vi "Intensity.vi"(1 "PSD[0]":dbl[](array[numeric])) -> (0 "Intensity":T1)   [LabVIEW 2013]
uses:
  <vilib>/Analysis/5stat.llb/RMS (DBL).vi
  <vilib>/Analysis/NI_AALPro.lvlib
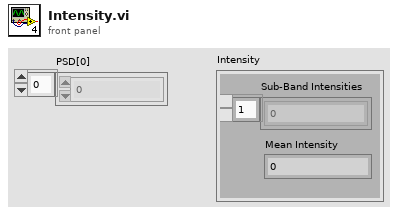
[diagram p1: front panel]
types:
  T1 = cluster{"Sub-Band Intensities":dbl[], "Mean Intensity":dbl}
  T2 = cluster{"1":dbl[], "2":dbl[], "3":dbl[], "4":dbl[], "5":dbl[], "6":dbl[], "7":dbl[]}
  T3 = cluster{"rms value":dbl, "rms value":dbl, "rms value":dbl, "rms value":dbl, "rms value":dbl, "rms value":dbl, "rms value":dbl}
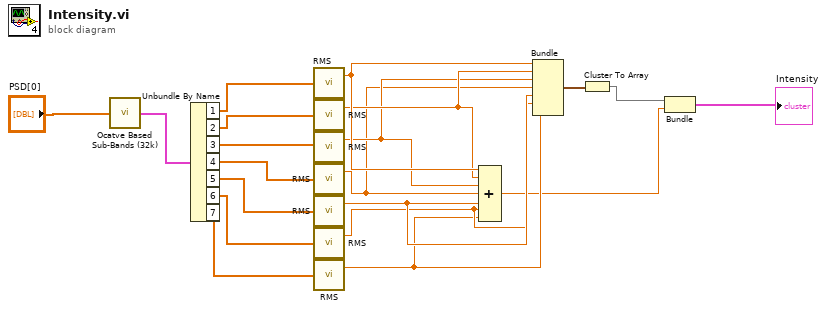
[diagram p0: block diagram]
diagram:
  n1 = call "Ocatve Based Sub-Bands (32k).vi"("Array"="PSD[0]") -> ("Sub-Band's"=w18:T2)
  n2 = Unbundle By Name(w18) -> ("1"=w17:dbl[], "2"=w16:dbl[], "3"=w15:dbl[], "4"=w14:dbl[], "5"=w13:dbl[], "6"=w12:dbl[], "7"=w11:dbl[])
  n3 = call-poly <vilib>:"RMS.vi"("X"=w17) -> ("rms value"=w10:dbl)  [unwired: 1 out]
  n4 = call-poly <vilib>:"RMS.vi"("X"=w16) -> ("rms value"=w9:dbl)  [unwired: 1 out]
  n5 = call-poly <vilib>:"RMS.vi"("X"=w15) -> ("rms value"=w8:dbl)  [unwired: 1 out]
  n6 = call-poly <vilib>:"RMS.vi"("X"=w14) -> ("rms value"=w7:dbl)  [unwired: 1 out]
  n7 = call-poly <vilib>:"RMS.vi"("X"=w13) -> ("rms value"=w6:dbl)  [unwired: 1 out]
  n8 = call-poly <vilib>:"RMS.vi"("X"=w12) -> ("rms value"=w5:dbl)  [unwired: 1 out]
  n9 = call-poly <vilib>:"RMS.vi"("X"=w11) -> ("rms value"=w4:dbl)  [unwired: 1 out]
  n10 = Compound Arithmetic op=ADD(w10, w9, w8, w7, w6, w5, w4) -> (w1:dbl)
  n11 = Bundle("rms value"=w10, "rms value"=w9, "rms value"=w8, "rms value"=w7, "rms value"=w6, "rms value"=w5, "rms value"=w4) -> (w3:T3)  [unwired: 1 in]
  n12 = Cluster To Array(cluster=w3) -> (array=w2:dbl[])
  n13 = Bundle(w2, w1) -> (→"Intensity":cluster{dbl[], dbl})  [unwired: 1 in]
